vi "LoadSetup.vi"(0 "select":enum16{"Init", "Read"}(ring)=enum."Read", 1 "section":string, 2 "key":string, 3 "default":string, 4 "error in (not an error)":errorcluster) -> (5 "error out":errorcluster={"status"=FALSE, "code"=0, "source"="Read File+ (string): Read File"}, 6 "value":string)   [LabVIEW 2010]
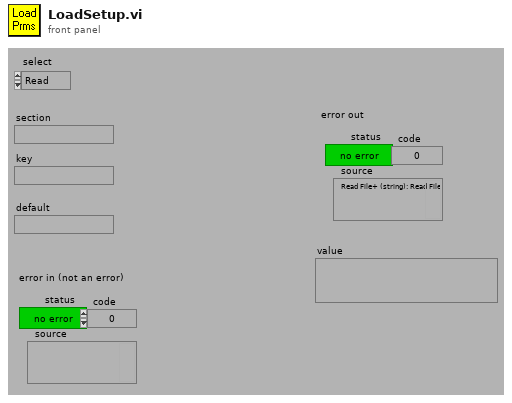
[diagram p1: front panel]
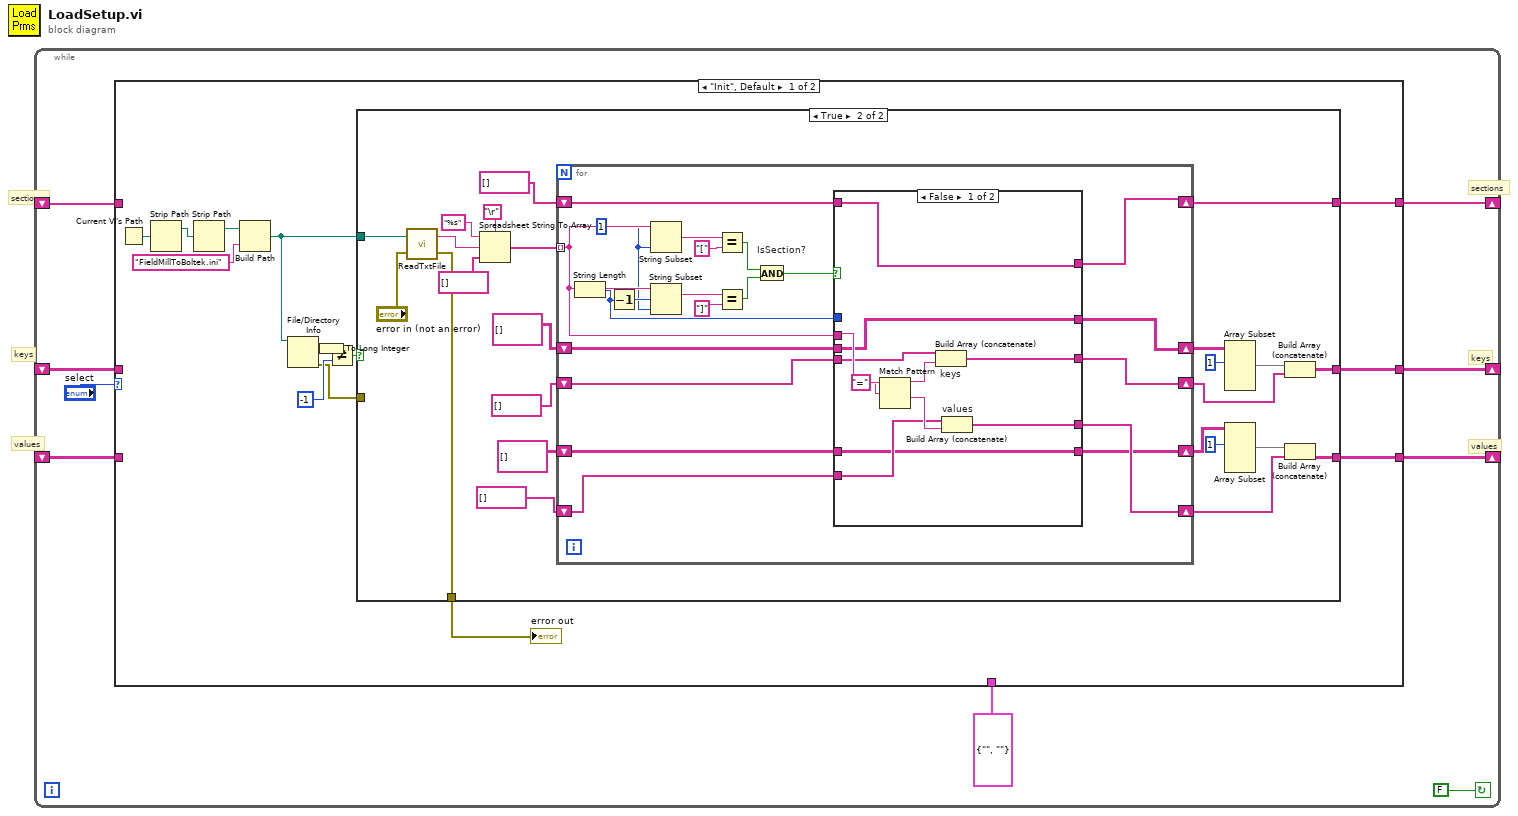
[diagram p0: block diagram]
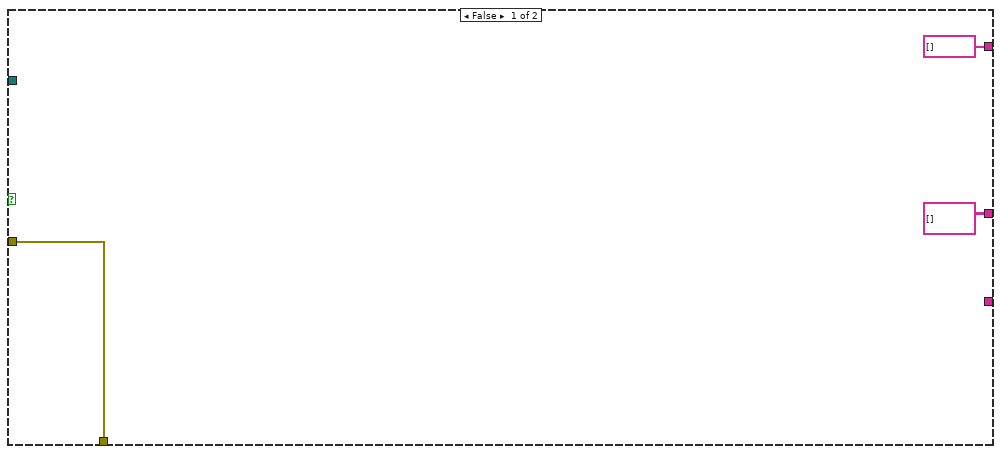
[diagram p2: hidden frame]
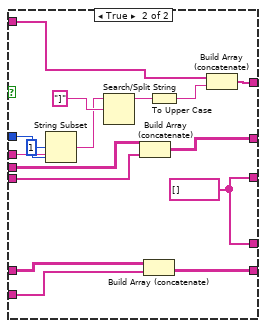
[diagram p3: hidden frame]
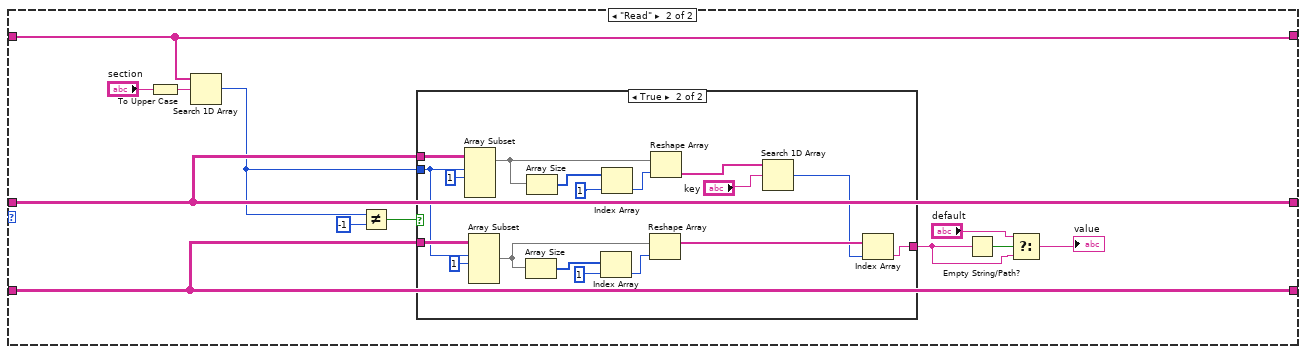
[diagram p4: hidden frame]
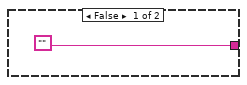
[diagram p5: hidden frame]
diagram:
  # "values"
  # "keys"
  # "sections"
  # "values"
  # "keys"
  # "sections"
  n1 = while {
    shift-left: _ -> [w1]
    shift-right: [w2] -> _
    shift-left: _ -> [w3]
    shift-right: [w4] -> _
    shift-left: _ -> [w5]
    shift-right: [w6] -> _
    stop <- FALSE continue-if-true
    n2 = case shown="\"Init\", Default" "select" {
      tunnel: cluster{"keys":string, "values":string} {"keys"="", "values"=""} ("SetupFile") -> [_ _]
      tunnel: [w19 w107] -> w6
      tunnel: w5 -> [_ w107]
      tunnel: [w18 w109] -> w4
      tunnel: w3 -> [_ w109]
      tunnel: [w17 w106] -> w2
      tunnel: w1 -> [_ w106]
      frame "Init", Default {
        n3 = Current VI's Path() -> (path=w23:path)
        n4 = Strip Path(path=w23) -> (stripped path=w22:path)  [unwired: 1 out]
        n5 = Strip Path(path=w22) -> (stripped path=w21:path)  [unwired: 1 out]
        n6 = Build Path(base path=w21, name or relative path="FieldMillToBoltek.ini") -> (appended path=w11:path)
        n7 = File/Directory Info(path=w11) -> (size=w10:i64, error out=w12:errorcluster)  [unwired: 1 in, 5 out]
        n8 = To Long Integer(number=w10) -> (32bit integer=w16:i32)
        n9 = Not Equal?(x=w16, y=-1) -> (x != y?=w14:bool)
        n10 = case shown="True" w14 {
          tunnel: [string[][] [] w41] -> w19
          tunnel: [string[] [] w40] -> w18
          tunnel: [_ w29] -> w17
          tunnel: w11 -> [_ w28]
          tunnel: [w24 w27] -> w13
          tunnel: w12 -> [w24 _]
          frame False {
          }
          frame True {
            n11 = call "ReadTxtFile.vi"("error in (not an error)"="error in (not an error)", "file path (dialog if empty)"=w28) -> ("error out"=w27:errorcluster, "line string"=w44:string)
            n12 = Spreadsheet String To Array(delimiter (Tab)="\r", format string="%s", spreadsheet string=w44, array type (2D Dbl)=string[] []) -> (array=w47:string[])
            n13 = for {
              tunnel: w47 -> [w65] mode=indexing
              shift-right: [w61] -> w40
              shift-left: string[] [] -> [w62]
              shift-right: [w54] -> w30
              shift-left: string[] [] -> [w55]
              shift-right: [w57] -> w36
              shift-left: string[][] [] -> [w58]
              shift-right: [w56] -> w35
              shift-left: string[] [] -> [w53]
              shift-right: [w52] -> w33
              shift-left: string[][] [] -> [w51]
              w64 = 1 ("length")
              n14 = String Length(string=w65) -> (length=w59:i32)
              n15 = Decrement(x=w59) -> (x-1=w68:i32)
              n16 = String Subset(string=w65, length (rest)=w64) -> (substring=w71:string)  [unwired: 1 in]
              n17 = String Subset(string=w65, offset (0)=w68, length (rest)=w64) -> (substring=w69:string)
              n18 = Equal?(x=w71, y="[") -> (x = y?=w67:bool)
              n19 = Equal?(x=w69, y="]" ("string")) -> (x = y?=w66:bool)
              n20 = And "IsSection?"(x=w67, y=w66) -> (x .and. y?=w63:bool)
              n21 = case shown="False" w63 {
                tunnel: w65 -> [w81 w94]
                tunnel: w62 -> [w82 w98]
                tunnel: [w82 w97] -> w61
                tunnel: w59 -> [_ w92]
                tunnel: [w79 w90] -> w57
                tunnel: w58 -> [w79 w84]
                tunnel: [w76 w88] -> w56
                tunnel: w55 -> [w75 w86]
                tunnel: [w74 w88] -> w54
                tunnel: w53 -> [w73 w87]
                tunnel: [w72 w85] -> w52
                tunnel: w51 -> [w72 w83]
                frame False {
                  n22 = Match Pattern(string=w81, regular expression="=") -> (before substring=w78:string, after substring=w77:string)  [unwired: 1 in, 2 out]
                  n23 = Build Array (concatenate) "keys"(w73, w78) -> (w76:string[])
                  n24 = Build Array (concatenate) "values"(w75, w77) -> (w74:string[])
                }
                frame True {
                  w88 = string[] []
                  n25 = String Subset(string=w94, offset (0)=1, length (rest)=w92) -> (substring=w91:string)
                  n26 = Search/Split String(string=w91, search string/char (-)="]") -> (substring before match=w96:string)  [unwired: 1 in, 2 out]
                  n27 = Build Array (concatenate)(w84, w87) -> (w90:string[][])
                  n28 = Build Array (concatenate)(w83, w86) -> (w85:string[][])
                  n29 = To Upper Case(1:w96) -> (0:w89:string)
                  n30 = Build Array (concatenate)(w98, w89) -> (w97:string[])
                }
              }
            }
            n31 = Array Subset(array=w36, index (row)=1) -> (w42:string[][])  [unwired: 3 in]
            n32 = Array Subset(array=w33, index (row)=1) -> (w34:string[][])  [unwired: 3 in]
            n33 = Build Array (concatenate)(w42, w35) -> (w41:string[][])
            n34 = Build Array (concatenate)(w34, w30) -> (w29:string[][])
          }
        }
        "error out" <- w13
      }
      frame "Read" {
        n35 = To Upper Case(1:"section") -> (0:w108:string)
        n36 = Search 1D Array(1D array=w109, element=w108) -> (index of element=w103:i32)  [unwired: 1 in]
        n37 = Not Equal?(x=w103, y=-1) -> (x != y?=w104:bool)
        n38 = case shown="True" w104 {
          tunnel: w107 -> [_ w123]
          tunnel: w106 -> [_ w121]
          tunnel: w103 -> [_ w120]
          tunnel: ["" w112] -> w100
          frame False {
          }
          frame True {
            n39 = Array Subset(array=w123, index (row)=w120, length (row)=1) -> (w128:string[][])  [unwired: 2 in]
            n40 = Array Subset(array=w121, index (row)=w120, length (row)=1) -> (w116:string[][])  [unwired: 2 in]
            n41 = Array Size(array=w116) -> (size(s)=w118:i32[])
            n42 = Array Size(array=w128) -> (size(s)=w127:i32[])
            n43 = Index Array(array=w118, index=1) -> (element=w115:i32)
            n44 = Index Array(array=w127, index=1) -> (element=w125:i32)
            n45 = Reshape Array(w116, w115) -> (w114:string[])
            n46 = Reshape Array(w128, w125) -> (w124:string[])
            n47 = Search 1D Array(1D array=w124, element="key") -> (index of element=w113:i32)  [unwired: 1 in]
            n48 = Index Array(array=w114, index=w113) -> (element=w112:string)
          }
        }
        n49 = Empty String/Path?(string/path=w100) -> (empty?=w102:bool)
        n50 = Select(t="default", s=w102, f=w100) -> (s? t:f=→"value":string)
      }
    }
  }
